vi "JTAG MSP430 RAM Test.vi"(11 "error in (no error)":errorcluster) -> (6 "Test Result":string, 15 "error out":errorcluster)   [LabVIEW 2010]
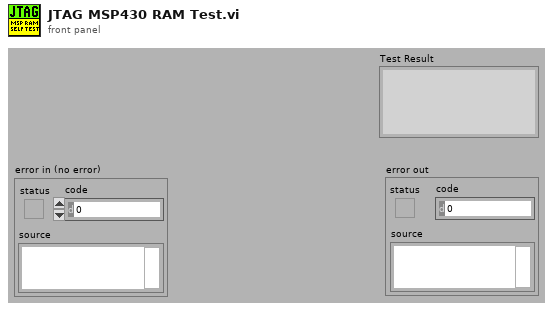
[diagram p1: front panel]
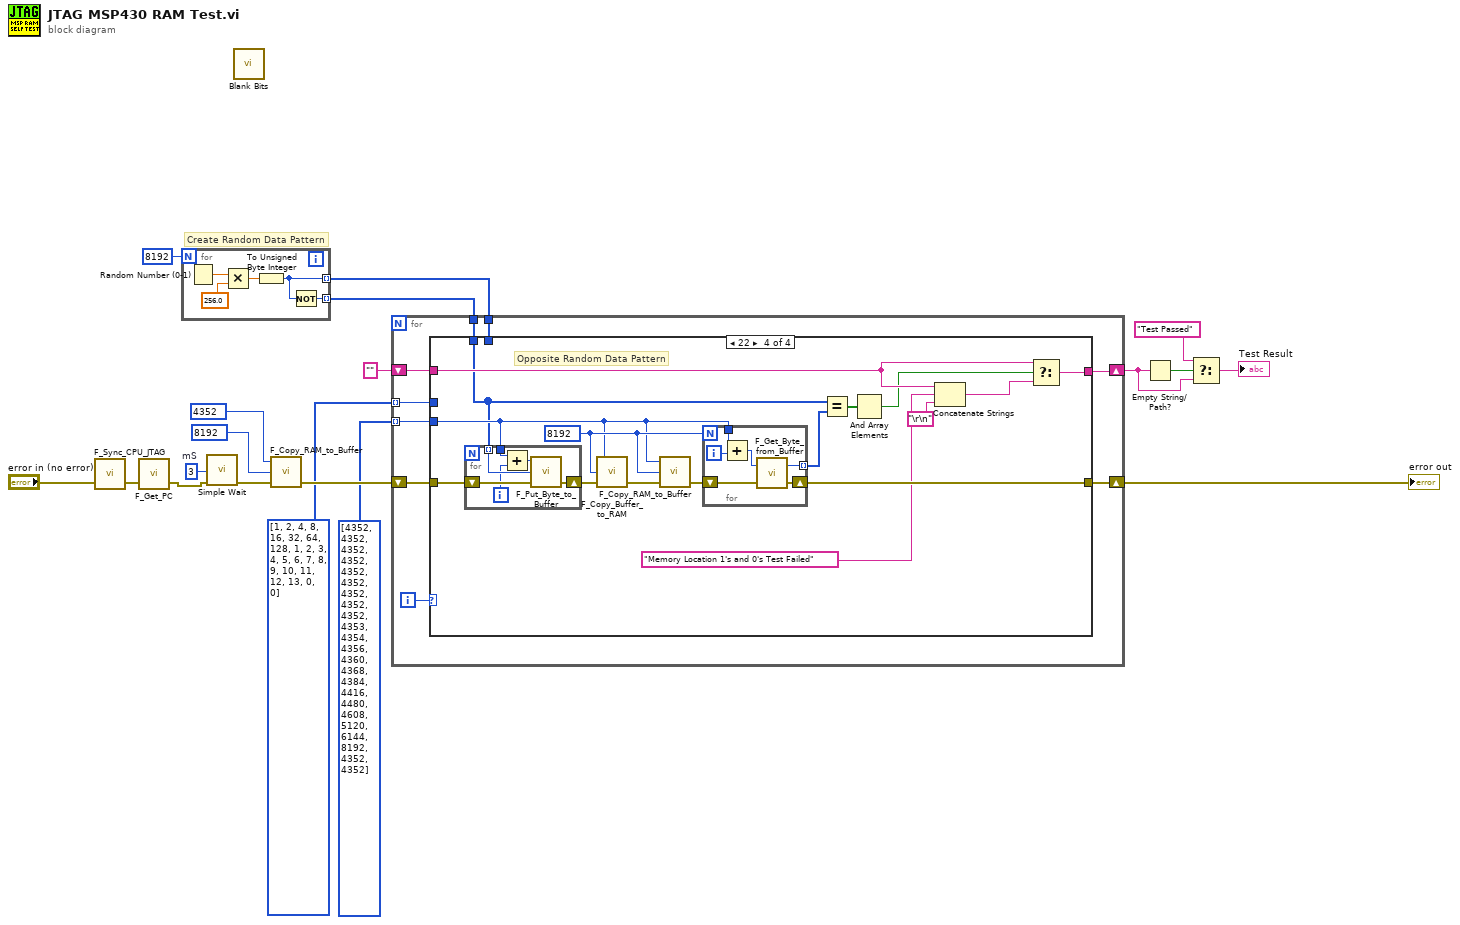
[diagram p0: block diagram]
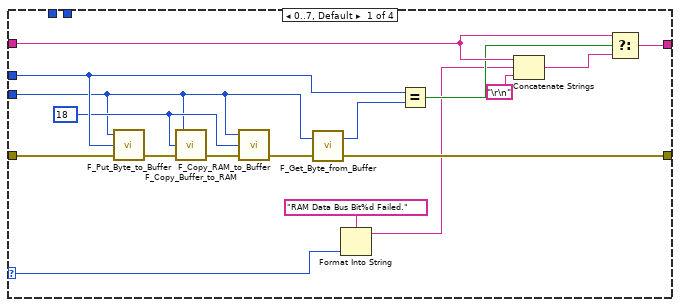
[diagram p2: hidden frame]
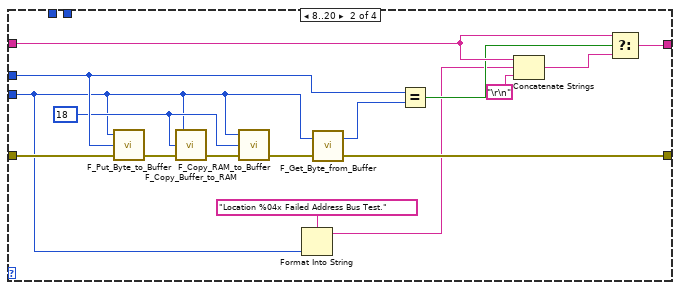
[diagram p3: hidden frame]
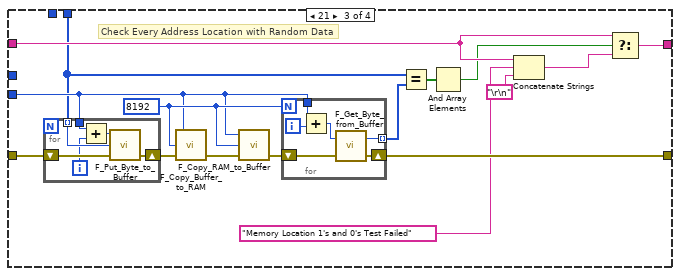
[diagram p4: hidden frame]
diagram:
  w11 = u32 3  # mS
  # "Create Random Data Pattern"
  n1 = call "F_Sync_CPU_JTAG.vi"("error in (no error)"="error in (no error)") -> ("error out"=w13:errorcluster)  [unwired: 1 in, 1 out]
  n2 = call "F_Get_PC.vi"("error in (no error)"=w13) -> ("error out"=w10:errorcluster)  [unwired: 1 in, 1 out]
  n3 = for {
    N: 8192 -> [_]
    tunnel: [w21] -> w2 mode=indexing
    tunnel: [w20] -> w1 mode=indexing
    n4 = Random Number (0-1)() -> (number: 0 to 1=w24:dbl)
    n5 = Multiply(x=w24, y=256.0) -> (x*y=w22:dbl)
    n6 = To Unsigned Byte Integer(number=w22) -> (unsigned 8bit integer=w21:u8)
    n7 = Not(x=w21) -> (.not. x?=w20:u8)
  }
  n8 = call "Simple Wait.vi"("mS"=w11, "error in"=w10) -> ("error out"=w9:errorcluster)  [unwired: 12 in, 1 out]
  n9 = call "Blank Bits.vi"() -> ()  [unwired: 14 in, 2 out]
  n10 = call "F_Copy_RAM_to_Buffer.vi"("error in (no error)"=w9, "Block size to be copied"=8192, "RAM start address"=4352) -> ("error out"=w8:errorcluster)  [unwired: 2 in]
  n11 = for {
    shift-right: [w32] -> w16
    shift-left: "" -> [w31]
    shift-right: [w30] -> w18
    shift-left: w8 -> [w33]
    tunnel: u8[] [1, 2, 4, 8, 16, 32, 64, 128, 1, 2, 3, 4, 5, 6, 7, 8, 9, 10, 11, 12, 13, 0, 0] -> [w28] mode=indexing
    tunnel: i32[] [4352, 4352, 4352, 4352, 4352, 4352, 4352, 4352, 4352, 4353, 4354, 4356, 4360, 4368, 4384, 4416, 4480, 4608, 5120, 6144, 8192, 4352, 4352] -> [w27] mode=indexing
    tunnel: w2 -> [w26]
    tunnel: w1 -> [w25]
    i -> [w29]
    n12 = case shown="22" w29 {
      selector: w29 -> [w35 _ _ _]
      tunnel: w33 -> [w42 w58 w74 w102]
      tunnel: [w38 w54 w72 w100] -> w30
      tunnel: [w50 w66 w82 w110] -> w32
      tunnel: w31 -> [w49 w65 w81 w109]
      tunnel: w28 -> [w40 w56 _ _]
      tunnel: w27 -> [w34 w51 w70 w98]
      tunnel: w26 -> [_ _ w69 _]
      tunnel: w25 -> [_ _ _ w96]
      frame 0..7, Default {
        w39 = 18
        n13 = call "F_Put_Byte_to_Buffer.vi"("error in (no error)"=w42, "New value"=w40, "Address of byte to be updated"=w34) -> ("error out"=w43:errorcluster)  [unwired: 2 in]
        n14 = call "F_Copy_Buffer_to_RAM.vi"("error in (no error)"=w43, "Block size to be copied"=w39, "Buffer start address"=w34) -> ("error out"=w44:errorcluster)  [unwired: 2 in]
        n15 = call "F_Copy_RAM_to_Buffer.vi"("error in (no error)"=w44, "Block size to be copied"=w39, "RAM start address"=w34) -> ("error out"=w45:errorcluster)  [unwired: 2 in]
        n16 = call "F_Get_Byte_from_Buffer.vi"("error in (no error)"=w45, "Address of byte to be read"=w34) -> ("error out"=w38:errorcluster, "Current value"=w41:u8)
        n17 = Format Into String(format string="RAM Data Bus Bit%d Failed." ("string"), w35) -> (resulting string=w36:string)  [unwired: 2 in, 1 out]
        n18 = Equal?(x=w40, y=w41) -> (x = y?=w46:bool)
        n19 = Concatenate Strings(w49, w36, "\r\n") -> (w48:string)
        n20 = Select(t=w49, s=w46, f=w48) -> (s? t:f=w50:string)
      }
      frame 8..20 {
        w55 = 18
        n21 = call "F_Put_Byte_to_Buffer.vi"("error in (no error)"=w58, "New value"=w56, "Address of byte to be updated"=w51) -> ("error out"=w59:errorcluster)  [unwired: 2 in]
        n22 = call "F_Copy_Buffer_to_RAM.vi"("error in (no error)"=w59, "Block size to be copied"=w55, "Buffer start address"=w51) -> ("error out"=w60:errorcluster)  [unwired: 2 in]
        n23 = call "F_Copy_RAM_to_Buffer.vi"("error in (no error)"=w60, "Block size to be copied"=w55, "RAM start address"=w51) -> ("error out"=w61:errorcluster)  [unwired: 2 in]
        n24 = Format Into String(format string="Location %04x Failed Address Bus Test." ("string"), w51) -> (resulting string=w52:string)  [unwired: 2 in, 1 out]
        n25 = call "F_Get_Byte_from_Buffer.vi"("error in (no error)"=w61, "Address of byte to be read"=w51) -> ("error out"=w54:errorcluster, "Current value"=w57:u8)
        n26 = Equal?(x=w56, y=w57) -> (x = y?=w62:bool)
        n27 = Concatenate Strings(w65, w52, "\r\n") -> (w64:string)
        n28 = Select(t=w65, s=w62, f=w64) -> (s? t:f=w66:string)
      }
      frame 21 {
        w71 = 8192
        # "Check Every Address Location with Random Data"
        n29 = for {
          tunnel: w70 -> [w90]
          shift-right: [w94] -> w75
          shift-left: w74 -> [w93]
          tunnel: w69 -> [w92] mode=indexing
          i -> [w89]
          n30 = Add(x=w90, y=w89) -> (x+y=w91:i32)
          n31 = call "F_Put_Byte_to_Buffer.vi"("error in (no error)"=w93, "New value"=w92, "Address of byte to be updated"=w91) -> ("error out"=w94:errorcluster)  [unwired: 2 in]
        }
        n32 = call "F_Copy_Buffer_to_RAM.vi"("error in (no error)"=w75, "Block size to be copied"=w71, "Buffer start address"=w70) -> ("error out"=w76:errorcluster)  [unwired: 2 in]
        n33 = call "F_Copy_RAM_to_Buffer.vi"("error in (no error)"=w76, "Block size to be copied"=w71, "RAM start address"=w70) -> ("error out"=w77:errorcluster)  [unwired: 2 in]
        n34 = for {
          N: w71 -> [_]
          tunnel: [w87] -> w73 mode=indexing
          tunnel: w70 -> [w85]
          shift-right: [w86] -> w72
          shift-left: w77 -> [w88]
          i -> [w84]
          n35 = Add(x=w85, y=w84) -> (x+y=w83:i32)
          n36 = call "F_Get_Byte_from_Buffer.vi"("error in (no error)"=w88, "Address of byte to be read"=w83) -> ("error out"=w86:errorcluster, "Current value"=w87:u8)
        }
        n37 = Equal?(x=w69, y=w73) -> (x = y?=w78:bool[])
        n38 = And Array Elements(Boolean array=w78) -> (logical AND=w68:bool)
        n39 = Concatenate Strings(w81, "Memory Location 1's and 0's Test Failed" ("string"), "\r\n") -> (w80:string)
        n40 = Select(t=w81, s=w68, f=w80) -> (s? t:f=w82:string)
      }
      frame 22 {
        w99 = 8192
        # "Opposite Random Data Pattern"
        n41 = for {
          tunnel: w98 -> [w118]
          shift-right: [w122] -> w103
          shift-left: w102 -> [w121]
          tunnel: w96 -> [w120] mode=indexing
          i -> [w117]
          n42 = Add(x=w118, y=w117) -> (x+y=w119:i32)
          n43 = call "F_Put_Byte_to_Buffer.vi"("error in (no error)"=w121, "New value"=w120, "Address of byte to be updated"=w119) -> ("error out"=w122:errorcluster)  [unwired: 2 in]
        }
        n44 = call "F_Copy_Buffer_to_RAM.vi"("error in (no error)"=w103, "Block size to be copied"=w99, "Buffer start address"=w98) -> ("error out"=w104:errorcluster)  [unwired: 2 in]
        n45 = call "F_Copy_RAM_to_Buffer.vi"("error in (no error)"=w104, "Block size to be copied"=w99, "RAM start address"=w98) -> ("error out"=w105:errorcluster)  [unwired: 2 in]
        n46 = for {
          N: w99 -> [_]
          tunnel: [w115] -> w101 mode=indexing
          tunnel: w98 -> [w113]
          shift-right: [w114] -> w100
          shift-left: w105 -> [w116]
          i -> [w112]
          n47 = Add(x=w113, y=w112) -> (x+y=w111:i32)
          n48 = call "F_Get_Byte_from_Buffer.vi"("error in (no error)"=w116, "Address of byte to be read"=w111) -> ("error out"=w114:errorcluster, "Current value"=w115:u8)
        }
        n49 = Equal?(x=w96, y=w101) -> (x = y?=w106:bool[])
        n50 = And Array Elements(Boolean array=w106) -> (logical AND=w97:bool)
        n51 = Concatenate Strings(w109, "Memory Location 1's and 0's Test Failed" ("string"), "\r\n") -> (w108:string)
        n52 = Select(t=w109, s=w97, f=w108) -> (s? t:f=w110:string)
      }
    }
  }
  "error out" <- w18
  n53 = Empty String/Path?(string/path=w16) -> (empty?=w17:bool)
  n54 = Select(t="Test Passed", s=w17, f=w16) -> (s? t:f=→"Test Result":string)
